vi "2 absolute_speed.vi"(1 "Wind Vector":cluster{"Wind R":dbl, "Wind Theta":dbl}, 2 "Boat Angle":dbl) -> (0 "Velocity":dbl)   [LabVIEW 2011]
doc: "This VI takes in a boat angle and a wind angle and returns the speed that the boat can achieve. This is a unitless speed which is only relative to other values returned by VI."
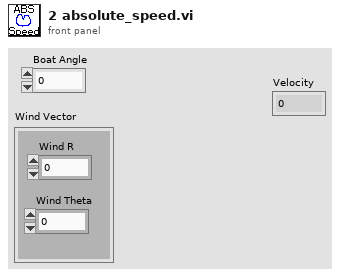
[diagram p1: front panel]
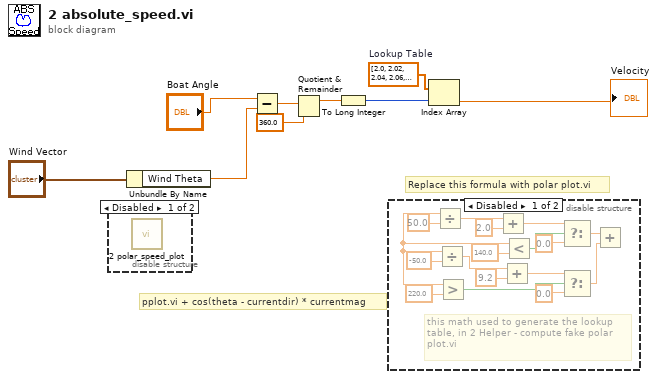
[diagram p0: block diagram]
diagram:
  w6 = dbl[] [2.0, 2.02, 2.04, 2.06, 2.08, 2.1, 2.12, 2.14, 2.16, 2.18, 2.2, 2.22, 2.24, 2.26, 2.2800000000000002, 2.3, 2.32, 2.34, 2.36, 2.38, 2.4, 2.42, 2.44, 2.46, 2.48, 2.5, 2.52, 2.54, 2.56, 2.58, 2.6, 2.62, 2.64, 2.66, 2.68, 2.7, 2.7199999999999998, 2.74, 2.76, 2.7800000000000002, 2.8, 2.82, 2.84, 2.86, 2.88, 2.9, 2.92, 2.94, 2.96, 2.98, 3.0, 3.02, 3.04, 3.06, 3.08, 3.1, 3.12, 3.1399999999999997, 3.16, 3.1799999999999997, 3.2, 3.2199999999999998, 3.24, 3.26, 3.2800000000000002, 3.3, 3.3200000000000003, 3.34, 3.3600000000000003, 3.38, 3.4, 3.42, 3.44, 3.46, 3.48, 3.5, 3.52, 3.54, 3.56, 3.58, 3.6, 3.62, 3.6399999999999997, 3.66, 3.6799999999999997, 3.7, 3.7199999999999998, 3.74, 3.76, 3.7800000000000002, 3.8, 3.8200000000000003, 3.84, 3.8600000000000003, 3.88, 3.9, 3.92, 3.94, 3.96, 3.98, 4.0, 4.02, 4.04, 4.0600000000000005, 4.08, 4.1, 4.12, 4.140000000000001, 4.16, 4.18, 4.2, 4.220000000000001, 4.24, 4.26, 4.279999999999999, 4.3, 4.32, 4.34, 4.359999999999999, 4.38, 4.4, 4.42, 4.4399999999999995, 4.46, 4.48, 4.5, 4.52, 4.54, 4.5600000000000005, 4.58, 4.6, 4.62, 4.640000000000001, 4.66, 4.68, 4.7, 4.720000000000001, 4.74, 4.76, 4.779999999999999, 0.0, 0.0, 0.0, 0.0, 0.0, 0.0, 0.0, 0.0, 0.0, 0.0, 0.0, 0.0, 0.0, 0.0, 0.0, 0.0, 0.0, 0.0, 0.0, 0.0, 0.0, 0.0, 0.0, 0.0, 0.0, 0.0, 0.0, 0.0, 0.0, 0.0, 0.0, 0.0, 0.0, 0.0, 0.0, 0.0, 0.0, 0.0, 0.0, 0.0, 0.0, 0.0, 0.0, 0.0, 0.0, 0.0, 0.0, 0.0, 0.0, 0.0, 0.0, 0.0, 0.0, 0.0, 0.0, 0.0, 0.0, 0.0, 0.0, 0.0, 0.0, 0.0, 0.0, 0.0, 0.0, 0.0, 0.0, 0.0, 0.0, 0.0, 0.0, 0.0, 0.0, 0.0, 0.0, 0.0, 0.0, 0.0, 0.0, 0.0, 0.0, 4.779999999999999, 4.759999999999999, 4.739999999999999, 4.719999999999999, 4.699999999999999, 4.68, 4.659999999999999, 4.64, 4.619999999999999, 4.6, 4.579999999999999, 4.56, 4.539999999999999, 4.52, 4.499999999999999, 4.4799999999999995, 4.459999999999999, 4.4399999999999995, 4.419999999999999, 4.3999999999999995, 4.379999999999999, 4.359999999999999, 4.339999999999999, 4.319999999999999, 4.299999999999999, 4.279999999999999, 4.259999999999999, 4.239999999999999, 4.219999999999999, 4.199999999999999, 4.18, 4.159999999999999, 4.14, 4.119999999999999, 4.1, 4.079999999999999, 4.06, 4.039999999999999, 4.02, 3.999999999999999, 3.9799999999999995, 3.959999999999999, 3.9399999999999995, 3.919999999999999, 3.8999999999999995, 3.879999999999999, 3.8599999999999994, 3.839999999999999, 3.8199999999999994, 3.799999999999999, 3.7799999999999994, 3.759999999999999, 3.7399999999999993, 3.719999999999999, 3.6999999999999993, 3.6799999999999997, 3.6599999999999993, 3.6399999999999997, 3.619999999999999, 3.5999999999999996, 3.579999999999999, 3.5599999999999996, 3.539999999999999, 3.5199999999999996, 3.499999999999999, 3.4799999999999995, 3.459999999999999, 3.4399999999999995, 3.419999999999999, 3.3999999999999995, 3.379999999999999, 3.3599999999999994, 3.339999999999999, 3.3199999999999994, 3.299999999999999, 3.2799999999999994, 3.259999999999999, 3.2399999999999993, 3.219999999999999, 3.1999999999999993, 3.1799999999999997, 3.1599999999999993, 3.1399999999999997, 3.119999999999999, 3.0999999999999996, 3.079999999999999, 3.0599999999999996, 3.039999999999999, 3.0199999999999996, 2.999999999999999, 2.9799999999999995, 2.959999999999999, 2.9399999999999995, 2.919999999999999, 2.8999999999999995, 2.879999999999999, 2.8599999999999994, 2.839999999999999, 2.8199999999999994, 2.799999999999999, 2.7799999999999994, 2.759999999999999, 2.7399999999999993, 2.719999999999999, 2.6999999999999993, 2.6799999999999997, 2.6599999999999993, 2.6399999999999997, 2.619999999999999, 2.5999999999999996, 2.579999999999999, 2.5599999999999996, 2.539999999999999, 2.5199999999999996, 2.499999999999999, 2.4799999999999995, 2.459999999999999, 2.4399999999999995, 2.419999999999999, 2.3999999999999995, 2.379999999999999, 2.3599999999999994, 2.339999999999999, 2.3199999999999994, 2.299999999999999, 2.2799999999999994, 2.259999999999999, 2.2399999999999993, 2.219999999999999, 2.1999999999999993, 2.1799999999999997, 2.1599999999999993, 2.1399999999999997, 2.119999999999999, 2.0999999999999996, 2.079999999999999, 2.0599999999999996, 2.039999999999999, 2.0199999999999996]  # Lookup Table
  # "Replace this formula with polar plot.vi"
  # "pplot.vi + cos(theta - currentdir) * currentmag"
  n1 = disable-structure shown="Disabled" {
    frame Disabled {
      n2 = call "2 polar_speed_plot.vi"() -> ()  [unwired: 2 in, 1 out]
    }
    frame Enabled {
    }
  }
  n3 = Unbundle By Name("Wind Vector") -> ("Wind Theta"=w7:dbl)
  n4 = Subtract(x="Boat Angle", y=w7) -> (x-y=w4:dbl)
  n5 = Quotient & Remainder(x=w4, y=360.0) -> (x-y*floor(x/y)=w2:dbl)  [unwired: 1 out]
  n6 = To Long Integer(number=w2) -> (32bit integer=w1:i32)
  n7 = disable-structure shown="Disabled" {
    frame Disabled {
      # "this math used to generate the lookup\ntable, in 2 Helper - compute fake polar\nplot.vi"
      n8 = Greater?(y=220.0) -> (x=w10:dbl, 0:w21:bool)
      n9 = Divide(x=w10, y=50.0) -> (x/y=w18:dbl)
      n10 = Divide(x=w10, y=-50.0) -> (x/y=w13:dbl)
      n11 = Add(x=w18, y=2.0) -> (x+y=w19:dbl)
      n12 = Add(x=w13, y=9.2) -> (x+y=w11:dbl)
      n13 = Less?(x=w10, y=140.0) -> (x < y?=w25:bool)
      n14 = Select(t=w19, s=w25, f=0.0) -> (s? t:f=w16:dbl)
      n15 = Select(t=w11, s=w21, f=0.0) -> (s? t:f=w15:dbl)
      n16 = Add(x=w16, y=w15) -> ()  [unwired: 1 out]
    }
    frame Enabled {
    }
  }
  n17 = Index Array(array=w6, index=w1) -> (element=→"Velocity":dbl)
